vi "Launch_File.vi"(5 "Flag":u16(ring)=1 items=["SW_HIDE", "SW_NORMAL", "SW_SHOWMINIMIZED", "SW_SHOWMAXIMIZED", "SW_SHOWNOACTIVATE", "SW_SHOW", "SW_MINIMIZE", "SW_SHOWMINNOACTIVE", "SW_SHOWNA", "SW_RESTORE", "SW_SHOWDEFAULT", "SW_FORCEMINIMIZE"], 6 "error in":errorcluster, 7 "Parameters":string, 8 "path":path=path "C:/test", 9 "Operation":T1(ring)) -> (4 "ERROR":bool)   [LabVIEW 2015]
uses:
  user32.dll
  shell32.dll
panel:
  out "output param":i32
  out "error out":errorcluster
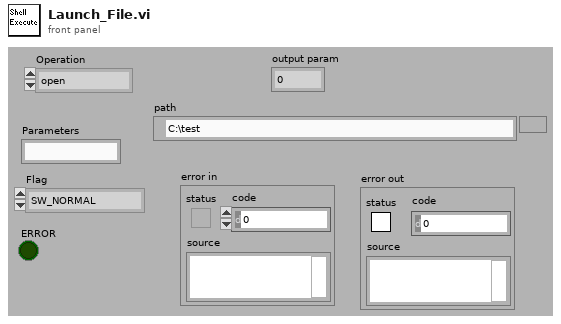
[diagram p1: front panel]
types:
  T1 = enum8{"open", "edit", "explore", "find", "print"}
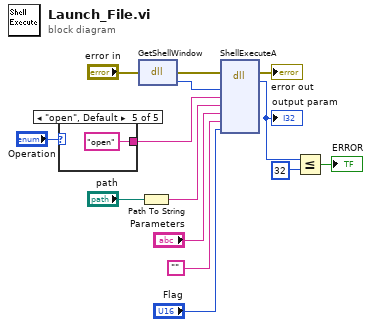
[diagram p0: block diagram]
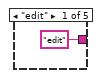
[diagram p2: hidden frame]
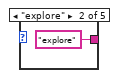
[diagram p3: hidden frame]
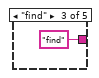
[diagram p4: hidden frame]
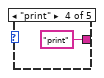
[diagram p5: hidden frame]
diagram:
  n1 = case shown="\"open\", Default" "Operation" {
    tunnel: ["edit" "explore" "find" "print" "open"] -> w11
    frame "edit" {
    }
    frame "explore" {
    }
    frame "find" {
    }
    frame "print" {
    }
    frame "open", Default {
    }
  }
  n2 = dll-call lib="user32.dll" fn="GetShellWindow"(error in="error in") -> (error out=w1:errorcluster, w14:u32)  [unwired: 2 in, 1 out]
  n3 = Path To String(path="path") -> (string=w10:string)
  n4 = dll-call lib="shell32.dll" fn="ShellExecuteA"(error in=w1, "hwnd"=w14, "lpOperation"=w11, "lpFile"=w10, "lpParameters"="Parameters", "lpDirectory"="", "nShowCmd"="Flag") -> (error out=→"error out":errorcluster, w6:i32)  [unwired: 5 in, 4 out]
  "output param" <- w6
  n5 = Less Or Equal?(x=w6, y=32) -> (x <= y?=→"ERROR":bool)
